vi "WriteVirtualStaveToFile.vi"() -> ()   [LabVIEW 2016]
uses:
  <vilib>/Utility/file.llb/Write Delimited Spreadsheet (DBL).vi
  Enum_TypeDef_TapeType.ctl
  Enum_TypeDef_FidMarkers.ctl
  Enum_TypeDef_Sensors.ctl
panel:
  in  "Distance between circular fid marks in Y [mm]":dbl=106.11
  in  "Distance between first locking point and first circular fid mark [mm]":dbl=54.735
  out "Module fiducials in the Stave's basis":T1(graph)=[{"Generated List of Module Coordinates"=[0.0, 280.05, 574.05, 868.05, 1162.05], "Generated List of Module Coordinates"=[0.0, 0.0, 0.0, 0.0, 0.0]}, {"Generated List of Module Coordinates"=[-4.719999999999999, 84.82000000000001, 84.82000000000001, -4.719999999999999, 93.28, 182.82000000000002, 182.82000000000002, 93.28, 191.28, 280.82, 280.82, 191.28, 289.28000000000003, 378.82, 378.82, 289.28000000000003, 387.28000000000003, 476.82, 476.82, 387.28000000000003, 485.28, 574.8199999999999, 574.8199999999999, 485.28, 583.28, 672.8199999999999, 672.8199999999999, 583.28, 681.28, 770.8199999999999, 770.8199999999999, 681.28, 779.28, 868.8199999999999, 868.8199999999999, 779.28, 877.28, 966.8199999999999, 966.8199999999999, 877.28, 975.28, 1064.82, 1064.82, 975.28, 1073.28, 1162.82, 1162.82, 1073.28, 1171.28, 1260.82, 1260.82, 1171.28], "Generated List of Module Coordinates"=[-19.901999999999994, -19.901999999999994, -109.44200000000001, -109.44200000000001, -19.901999999999994, -19.901999999999994, -109.44200000000001, -109.44200000000001, -19.901999999999994, -19.901999999999994, -109.44200000000001, -109.44200000000001, -19.901999999999994, -19.901999999999994, -109.44200000000001, -109.44200000000001, -19.901999999999994, -19.901999999999994, -109.44200000000001, -109.44200000000001, -19.901999999999994, -19.901999999999994, -109.44200000000001, -109.44200000000001, -19.901999999999994, -19.901999999999994, -109.44200000000001, -109.44200000000001, -19.901999999999994, -19.901999999999994, -109.44200000000001, -109.44200000000001, -19.901999999999994, -19.901999999999994, -109.44200000000001, -109.44200000000001, -19.901999999999994, -19.901999999999994, -109.44200000000001, -109.44200000000001, -19.901999999999994, -19.901999999999994, -109.44200000000001, -109.44200000000001, -19.901999999999994, -19.901999999999994, -109.44200000000001, -109.44200000000001, -19.901999999999994, -19.901999999999994, -109.44200000000001, -109.44200000000001]}, {"Generated List of Module Coordinates"=[40.050000000000004, 138.05, 236.05, 334.05, 432.05, 530.05, 628.05, 726.05, 824.05, 922.05, 1020.05, 1118.05, 1216.05], "Generated List of Module Coordinates"=[-64.672, -64.672, -64.672, -64.672, -64.672, -64.672, -64.672, -64.672, -64.672, -64.672, -64.672, -64.672, -64.672]}]
  in  "Stereo Angle [mrad]":dbl format="%#_13g"
  in  "N Modules":i32=13
  in  "Sensor Pattern":T2=enum."ATLAS12"
  in  "Module fiducial marker":T3=enum."KaptonSpacers"
  in  "Tape Type":T4=enum."Axial (Sutcliffe NP49-01-100 01-Mar-16)"
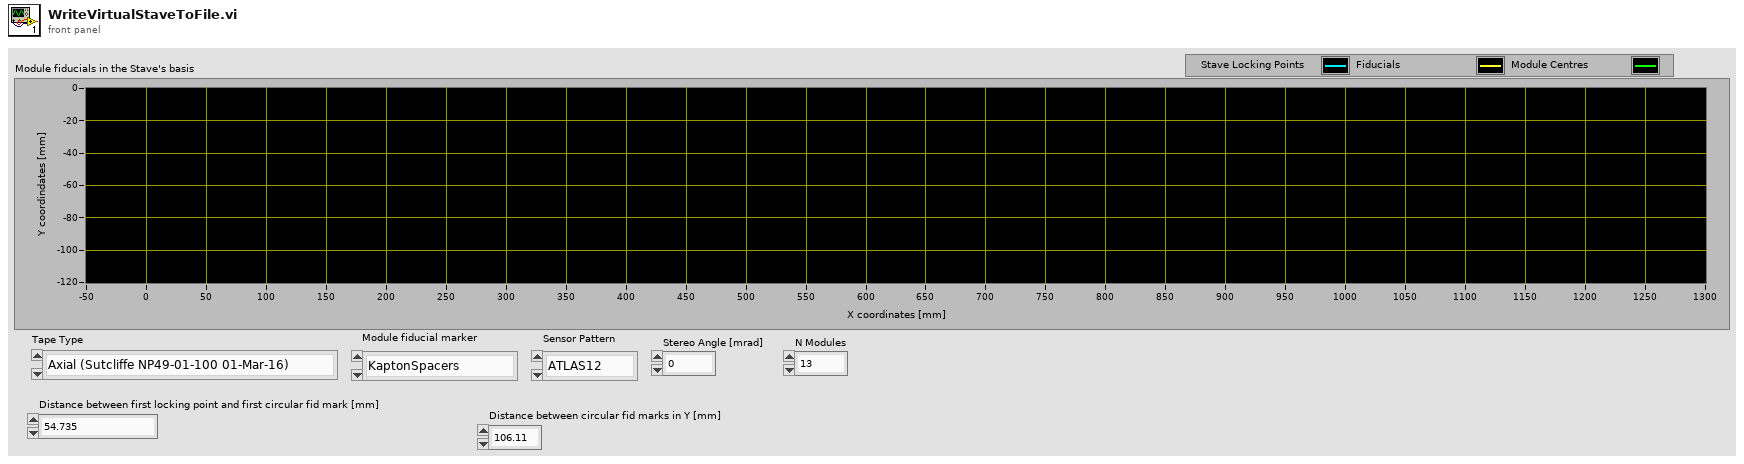
[diagram p1: front panel]
types:
  T1 = cluster{"Generated List of Module Coordinates":dbl[], "Generated List of Module Coordinates":dbl[]}[]
  T2 = typedef "Enum_TypeDef_Sensors.ctl" = enum16{"ATLAS07", "ATLAS12", "ATLAS12Slim", "ATLAS17LS"}
  T3 = typedef "Enum_TypeDef_FidMarkers.ctl" = enum16{"Mark B", "Mark C", "Strip Corner", "Mark I (Slim/17)", "Mark E (Slim/17)", "Mark F (Slim/17)", "Mark G (Slim/17)", "Mark A (12)", "KaptonSpacers"}
  T4 = typedef "Enum_TypeDef_TapeType.ctl" = enum16{"Right stereo", "Left stereo", "Stereo (Sutcliffe NP49-01-100 01-Mar-16)", "Axial (Sutcliffe NP49-01-100 01-Mar-16)"}
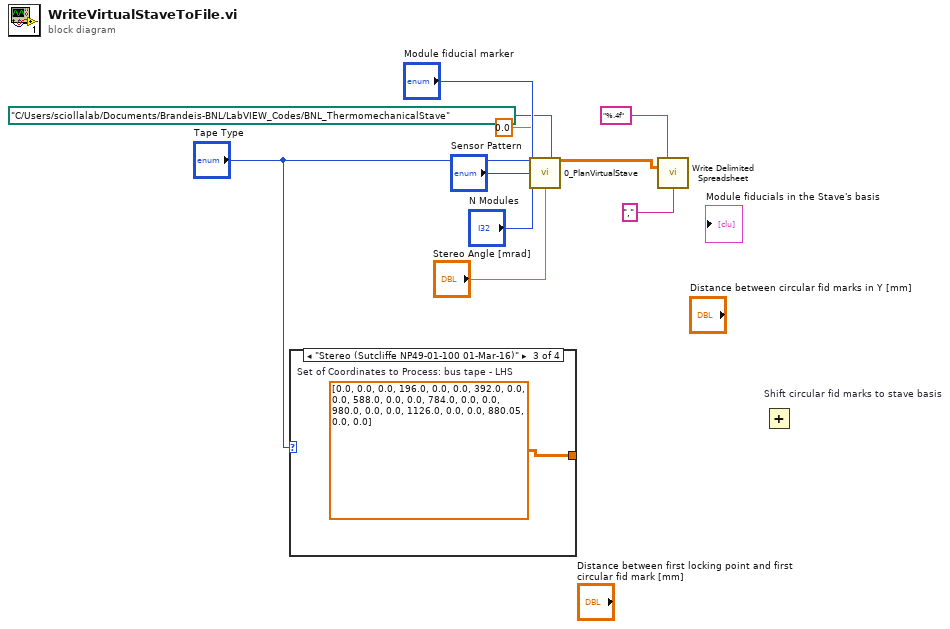
[diagram p0: block diagram]
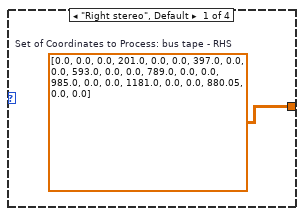
[diagram p2: hidden frame]
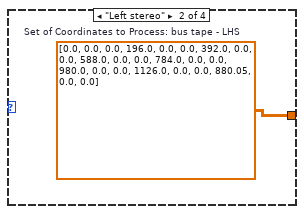
[diagram p3: hidden frame]
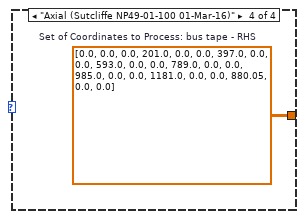
[diagram p4: hidden frame]
diagram:
  n1 = case shown="\"Stereo (Sutcliffe NP49-01-100 01-Mar-16)\"" "Tape Type" {
    tunnel: [w11 w12 w13 w14] -> _
    frame "Right stereo", Default {
      w11 = dbl[][] [[0.0, 0.0, 0.0], [201.0, 0.0, 0.0], [397.0, 0.0, 0.0], [593.0, 0.0, 0.0], [789.0, 0.0, 0.0], [985.0, 0.0, 0.0], [1181.0, 0.0, 0.0], [880.05, 0.0, 0.0]]  # Set of Coordinates to Process: bus tape - RHS
    }
    frame "Left stereo" {
      w12 = dbl[][] [[0.0, 0.0, 0.0], [196.0, 0.0, 0.0], [392.0, 0.0, 0.0], [588.0, 0.0, 0.0], [784.0, 0.0, 0.0], [980.0, 0.0, 0.0], [1126.0, 0.0, 0.0], [880.05, 0.0, 0.0]]  # Set of Coordinates to Process: bus tape - LHS
    }
    frame "Stereo (Sutcliffe NP49-01-100 01-Mar-16)" {
      w13 = dbl[][] [[0.0, 0.0, 0.0], [196.0, 0.0, 0.0], [392.0, 0.0, 0.0], [588.0, 0.0, 0.0], [784.0, 0.0, 0.0], [980.0, 0.0, 0.0], [1126.0, 0.0, 0.0], [880.05, 0.0, 0.0]]  # Set of Coordinates to Process: bus tape - LHS
    }
    frame "Axial (Sutcliffe NP49-01-100 01-Mar-16)" {
      w14 = dbl[][] [[0.0, 0.0, 0.0], [201.0, 0.0, 0.0], [397.0, 0.0, 0.0], [593.0, 0.0, 0.0], [789.0, 0.0, 0.0], [985.0, 0.0, 0.0], [1181.0, 0.0, 0.0], [880.05, 0.0, 0.0]]  # Set of Coordinates to Process: bus tape - RHS
    }
  }
  n2 = call "0_PlanVirtualStave.vi"("Tape Type"="Tape Type", "Code path"=path "C:/Users/sciollalab/Documents/Brandeis-BNL/LabVIEW_Codes/BNL_ThermomechanicalStave", "Module fiducial marker"="Module fiducial marker", "Sensor Pattern"="Sensor Pattern", "N Modules"="N Modules", "Working height [mm]"=0.0, "Stereo Angle [mrad]"="Stereo Angle [mrad]") -> ("Stave Basis: Coordinates of Fiducials on Modules"=w4:dbl[][])  [unwired: 6 in, 2 out]
  n3 = call-poly <vilib>:"Write Delimited Spreadsheet.vi"("format (%.3f)"="%.4f", "2D data"=w4, "delimiter (\\t)"="," ("delimiter (\\t)")) -> ()  [unwired: 11 in, 2 out]
  n4 = Add "Shift circular fid marks to stave basis"() -> ()  [unwired: 2 in, 1 out]
